vi "Write wait multiplier.vi"(8 "error in (no error)":errorcluster, 10 "wait multiplier":sgl, 11 "RTU Data Unit in":refnum<class "RTU Data Unit.lvclass">) -> (0 "error out":errorcluster, 3 "RTU Data Unit out":refnum<class "RTU Data Unit.lvclass">)   [LabVIEW 2013, in "Modbus Library - Advance.lvlib" / "RTU Data Unit.lvclass"]
uses:
  RTU Data Unit.lvclass
  RTU Data Unit.lvclass/RTU Data Unit.ctl
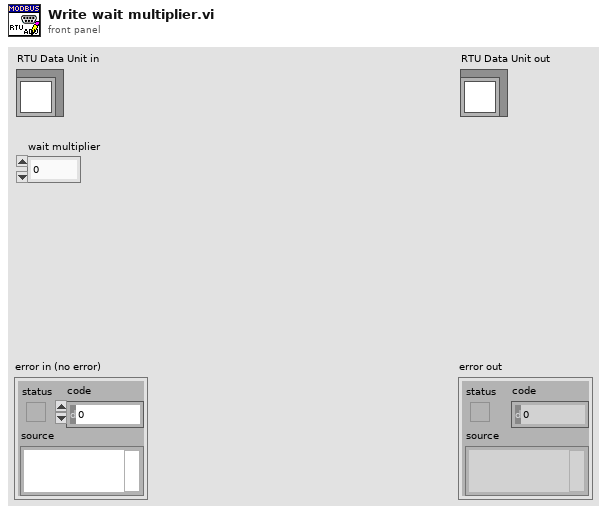
[diagram p1: front panel]
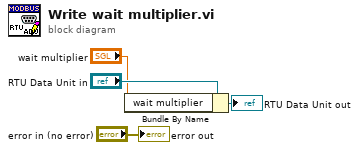
[diagram p0: block diagram]
diagram:
  n1 = Bundle By Name(cluster="RTU Data Unit in", "wait multiplier"="wait multiplier") -> (→"RTU Data Unit out":refnum<class "RTU Data Unit.lvclass">)
  "error out" <- "error in (no error)"
